vi "Utility_Pad_String.vi"(8 "error in (no error)":errorcluster, 9 "Null Terminate?(T)":bool=TRUE, 10 "Target Length":i32, 11 "String in":string) -> (0 "error out":errorcluster, 2 "Length out":i32, 3 "result string":string)   [LabVIEW 2021]
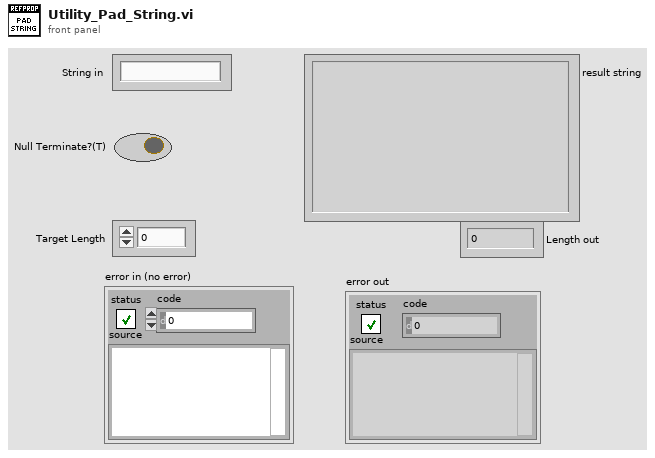
[diagram p1: front panel]
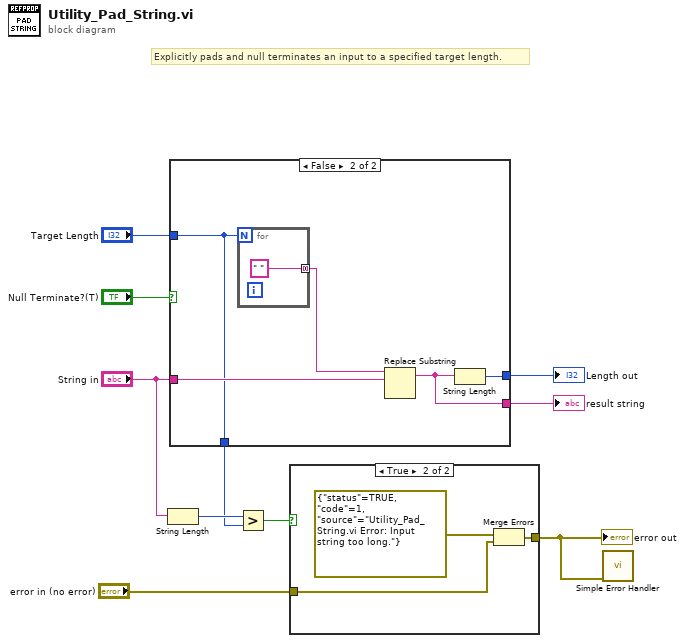
[diagram p0: block diagram]
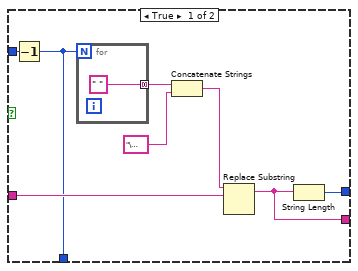
[diagram p2: hidden frame]
diagram:
  # "Explicitly pads and null terminates an input to a specified target length."
  n1 = String Length(string="String in") -> (length=w8:i32)
  n2 = case shown="False" "Null Terminate?(T)" {
    tunnel: [w18 w24] -> w10
    tunnel: [w14 w23] -> w9
    tunnel: "String in" -> [w13 w22]
    tunnel: "Target Length" -> [w12 w21]
    tunnel: [w11 w21] -> w2
    frame True {
      n3 = Decrement(x=w12) -> (x-1=w11:i32)
      n4 = for {
        N: w11 -> [_]
        tunnel: [" "] -> w15 mode=concatenating
      }
      n5 = Concatenate Strings(w15, "\u0000" ("string")) -> (w17:string)
      n6 = Replace Substring(4:w13, 5:w17) -> (1:w14:string)  [unwired: 2 in, 1 out]
      n7 = String Length(string=w14) -> (length=w18:i32)
    }
    frame False {
      n8 = for {
        N: w21 -> [_]
        tunnel: [" "] -> w20 mode=concatenating
      }
      n9 = Replace Substring(4:w22, 5:w20) -> (1:w23:string)  [unwired: 2 in, 1 out]
      n10 = String Length(string=w23) -> (length=w24:i32)
    }
  }
  "Length out" <- w10
  "result string" <- w9
  n11 = Greater?(x=w8, y=w2) -> (0:w6:bool)
  n12 = case shown="True" w6 {
    tunnel: "error in (no error)" -> [w26 w28]
    tunnel: [w26 w27] -> w3
    frame False {
    }
    frame True {
      n13 = Merge Errors(errorcluster {"status"=TRUE, "code"=1, "source"="Utility_Pad_String.vi Error: Input string too long."} ("error constant"), w28) -> (w27:errorcluster)
    }
  }
  "error out" <- w3
  n14 = call <vilib>:"Simple Error Handler.vi"("error in (no error)"=w3) -> ()  [unwired: 4 in, 5 out]
